vi "test_DL120115FPGA.vi"() -> ()   [LabVIEW 2010, in "FPGAWrapperDL090211Galvo_grabber.lvclass"]
uses:
  FPGAWrapperDL090211Galvo_grabber.lvclass
  common_typedefs/channels_cluster.ctl
  common_typedefs/gate_parameters_cluster.ctl
  common/classes/ErrorController/ErrorController/ErrorController.lvclass
  common/classes/ErrorController/ErrorController/class_data.vi
panel:
  in  "triggered?":bool
  out "samples read":i32
  in  "gate 1 settings":T1
  in  "channel offsets":T2
  out "error controller loaded?":bool=TRUE
  out "pixel dwell time":dbl[unit]
  out "timed out?":bool
  in  "timeout (ms)":i32=500
  out "DAQ loop counter":i32
  out "channel data block":dbl[][](graph)
  in  "number of channels":i32=3
  in  "block size":i32=10000
  out "DL090211FPGAWrapper out":refnum<class "FPGAWrapperDL090211Galvo_grabber.lvclass">
  in  "number of pixels":i64=1000000000
  in  "iterations per pixel":i32=250
  in  "run button":bool
  in  "stop":bool
  in  "create button":bool
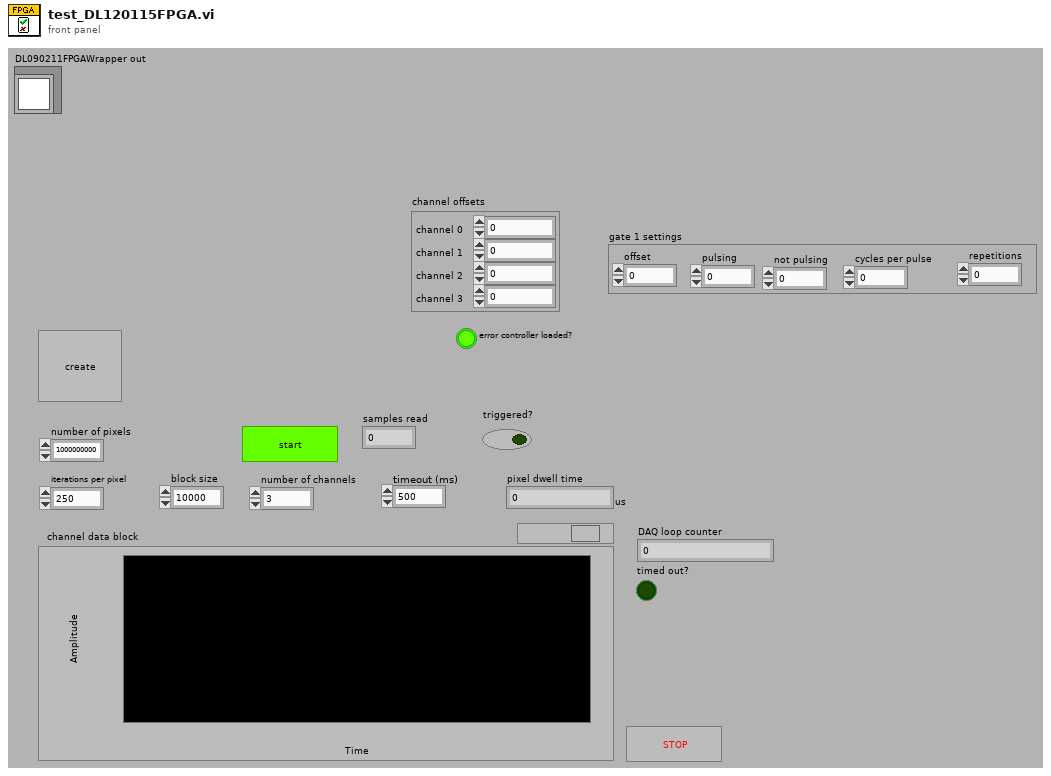
[diagram p1: front panel]
types:
  T1 = typedef "gate_parameters_cluster.ctl" = cluster{"offset":i64, "pulsing":i64, "not pulsing":i64, "cycles per pulse":i64, "repetitions":i64}
  T2 = typedef "channels_cluster.ctl" = cluster{"channel 0":u32, "channel 1":u32, "channel 2":u32, "channel 3":u32}
  T3 = typedef "pixel_raw_data_array.ctl" = dbl[][]
  T4 = typedef "plugin_specification.ctl" = cluster{"class path":string, "configuration":string, "label":string, "settings name":string}
  T5 = typedef "XComponentSpecification.xctl/data.ctl" = cluster{"class path":string, "configuration":string, "label":string, "settings name":string}
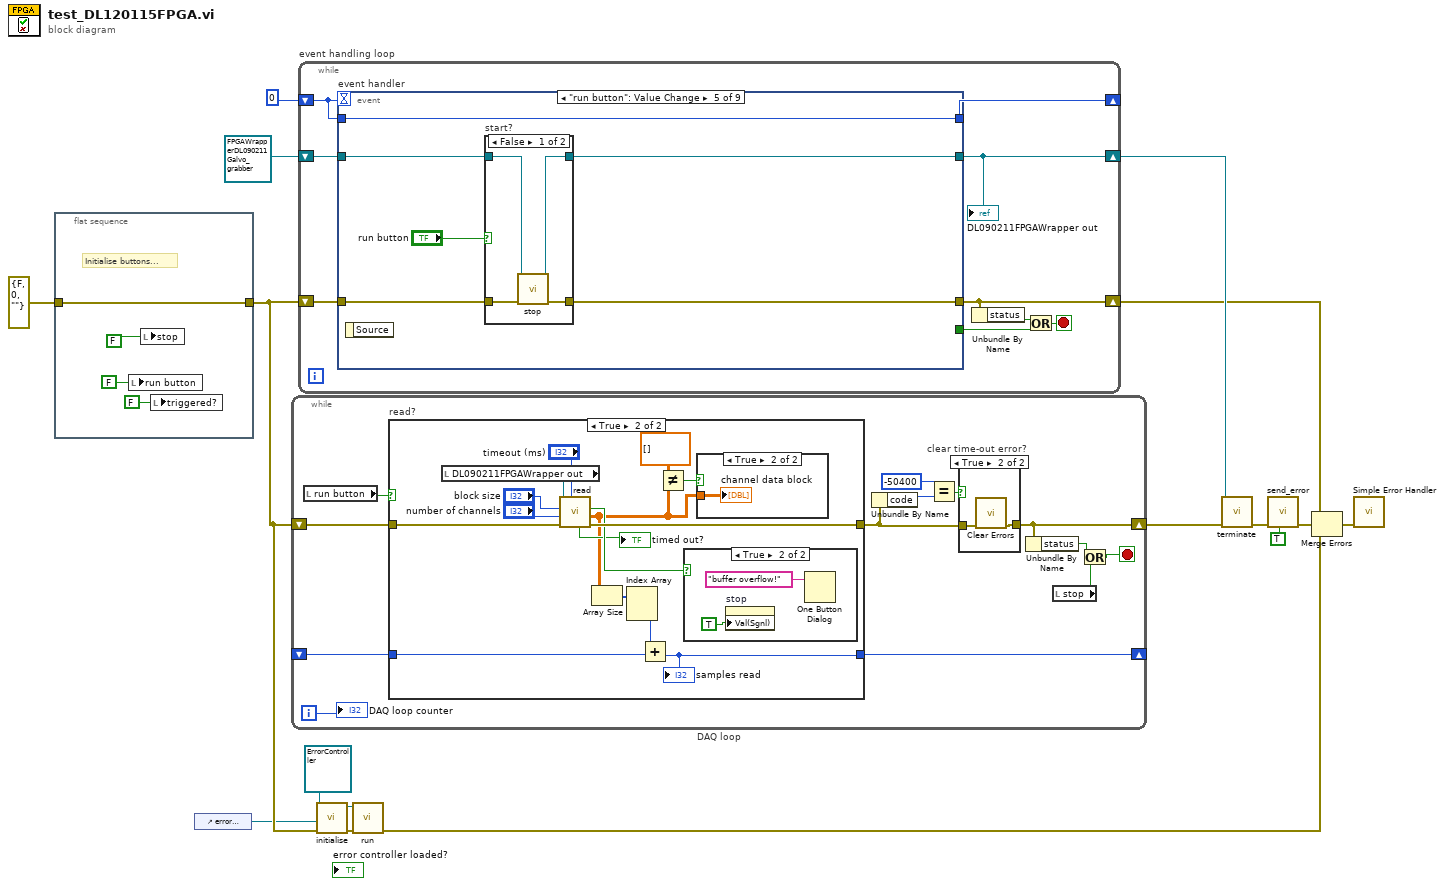
[diagram p0: block diagram]
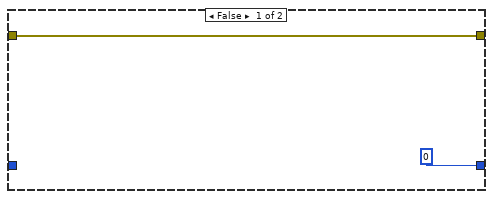
[diagram p3: hidden frame]
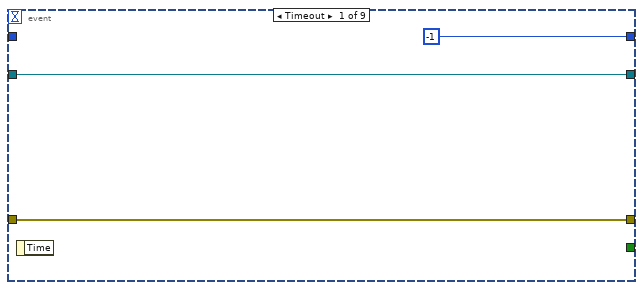
[diagram p6: hidden frame]
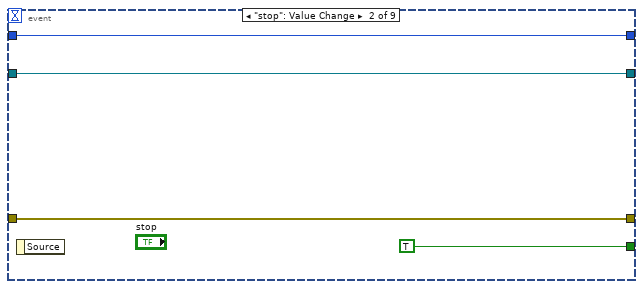
[diagram p7: hidden frame]
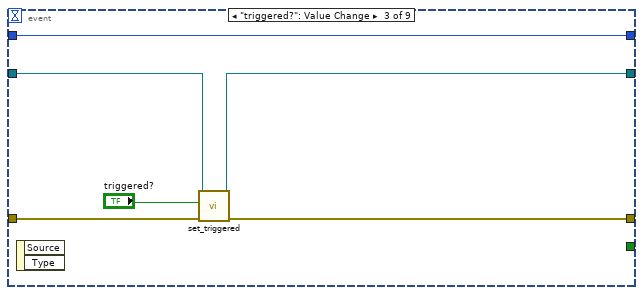
[diagram p8: hidden frame]
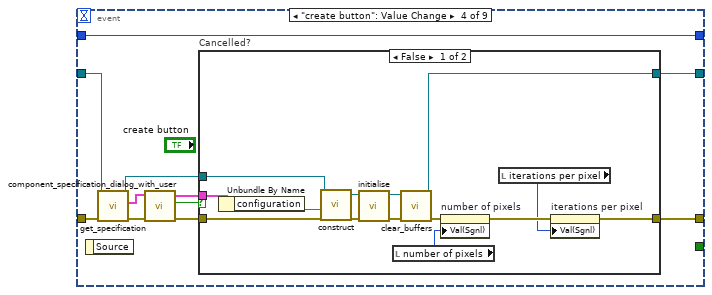
[diagram p9: hidden frame]
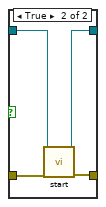
[diagram p11: hidden frame]
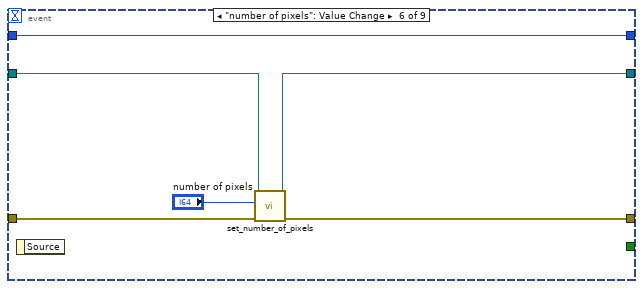
[diagram p12: hidden frame]
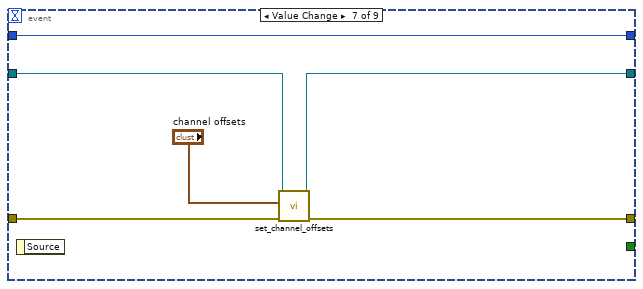
[diagram p13: hidden frame]
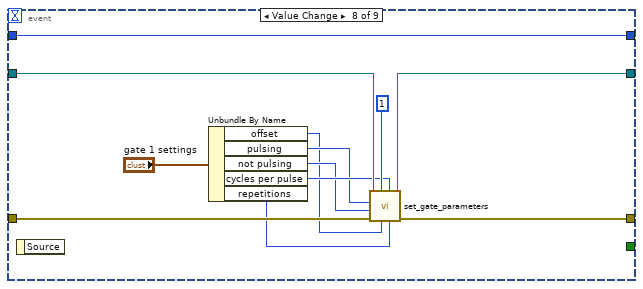
[diagram p14: hidden frame]
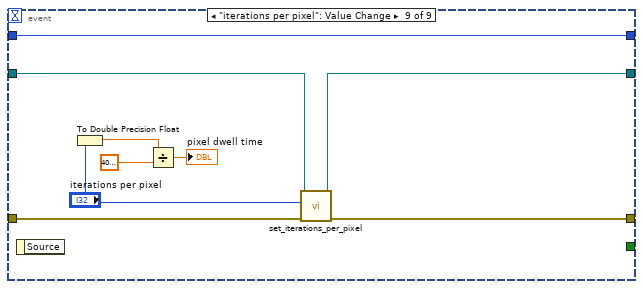
[diagram p15: hidden frame]
diagram:
  n1 = flat-sequence {
    tunnel: errorcluster {"status"=FALSE, "code"=0, "source"=""} ("error in (no error)") -> [w20]
    tunnel: [w20] -> w6
    frame #0 {
      # "Initialise buttons..."
      n2 = local write "run button"(FALSE ("run button")) -> ()
      n3 = local write "stop"(FALSE) -> ()
      n4 = local write "triggered?"(FALSE ("triggered?")) -> ()
    }
  }
  n5 = control-ref of="error controller loaded?"() -> (w1:refnum<vi>)
  n6 = while "DAQ loop" {
    shift-right: [w27] -> w13
    shift-left: w6 -> [w33]
    shift-right: [w21] -> _
    shift-left: _ -> [w22]
    i -> [w23]
    stop <- w24 stop-if-true
    n7 = local read "run button"() -> (w32:bool)
    n8 = case "read?" shown="True" w32 {
      tunnel: w33 -> [w38 w53]
      tunnel: [w38 w52] -> w29
      tunnel: w22 -> [_ w43]
      tunnel: [0 w40] -> w21
      frame False {
      }
      frame True {
        n9 = local read "DL090211FPGAWrapper out"() -> (w51:refnum<class "FPGAWrapperDL090211Galvo_grabber.lvclass">)
        n10 = call-dynamic "read.vi"("timeout (ms)"="timeout (ms)", "error in (no error)"=w53, "number of channels"="number of channels", "block size"="block size", "FPGAWrapperDL090211Galvo in"=w51) -> ("error out"=w52:errorcluster, "channels raw data block"=w42:T3, "FIFO full?"=w46:bool, "timed out?"=→"timed out?":bool)  [unwired: 3 out]
        n11 = Array Size(array=w42) -> (size(s)=w41:i32[])
        n12 = Index Array(array=w41) -> (element #2=w39:i32)  [unwired: 2 in, 1 out]
        n13 = Add(x=w39, y=w43) -> (x+y=w40:i32)
        "samples read" <- w40
        n14 = Not Equal?(x=dbl[][] [], y=w42) -> (x != y?=w48:bool)
        n15 = case shown="True" w46 {
          frame False {
          }
          frame True {
            n16 = property on="stop" class="Bool (strict)"("Val(Sgnl)"=TRUE) -> ()  [unwired: 2 in, 2 out]
            n17 = One Button Dialog(message="buffer overflow!") -> ()  [unwired: 1 in, 1 out]
          }
        }
        n18 = case shown="True" w48 {
          tunnel: w42 -> [_ w56]
          frame False {
          }
          frame True {
            "channel data block" <- w56
          }
        }
      }
    }
    n19 = Unbundle By Name(w29) -> ("code"=w31:i32)
    n20 = Equal?(x=-50400, y=w31) -> (x = y?=w28:bool)
    n21 = case "clear time-out error?" shown="True" w28 {
      tunnel: w29 -> [w34 w36]
      tunnel: [w34 w35] -> w27
      frame False {
      }
      frame True {
        n22 = call <vilib>:"Clear Errors.vi"("error in (no error)"=w36) -> ("error out"=w35:errorcluster)  [unwired: 6 out]
      }
    }
    n23 = Unbundle By Name(w27) -> ("status"=w26:bool)
    n24 = local read "stop"() -> (w25:bool)
    n25 = Or(x=w26, y=w25) -> (x .or. y?=w24:bool)
    "DAQ loop counter" <- w23
  }
  n26 = while "event handling loop" {
    shift-right: [w60] -> w11
    shift-left: w6 -> [w65]
    shift-right: [w63] -> _
    shift-left: 0 -> [w64]
    shift-right: [w61] -> w12
    shift-left: refnum<class "FPGAWrapperDL090211Galvo_grabber.lvclass"> refnum ("DL090211FPGAWrapper.lvclass") -> [w62]
    stop <- w57 stop-if-true
    n27 = event "event handler" shown="[4] \"run button\": Value Change" {
      selector: _ -> [_ _ _ _ _ _ _ _ _]
      dyn-events: _ -> [_ _ _ _ _ _ _ _ _]
      timeout: w64 -> [_ _ _ _ _ _ _ _ _]
      tunnel: [w66 w69 w76 w88 w107 w123 w129 w141 w150] -> w60
      tunnel: w65 -> [w66 w69 w77 w85 w110 w124 w130 w142 w151]
      tunnel: w64 -> [_ w72 w78 w89 w111 w125 w131 w143 w152]
      tunnel: [-1 w72 w78 w89 w111 w125 w131 w143 w152] -> w63
      tunnel: [_ TRUE _ _ _ _ _ _ _] -> w58
      tunnel: [w67 w70 w74 w80 w108 w121 w126 w139 w148] -> w61
      tunnel: w62 -> [w67 w70 w75 w83 w109 w122 w127 w140 w149]
      event Timeout {
        n28 = event-data() -> ()  [unwired: 2 out]
      }
      event "stop": Value Change {
        n29 = event-data() -> ()  [unwired: 2 out]
      }
      event "triggered?": Value Change {
        n30 = event-data() -> ()  [unwired: 3 out]
        n31 = call-dynamic "set_triggered.vi"("error in (no error)"=w77, "triggered?"="triggered?", "FPGAWrapperDL090211Galvo in"=w75) -> ("error out"=w76:errorcluster, "FPGAWrapperDL090211Galvo out"=w74:refnum<class "FPGAWrapperDL090211Galvo_grabber.lvclass">)  [unwired: 7 in]
      }
      event "create button": Value Change {
        n32 = event-data() -> ()  [unwired: 2 out]
        n33 = call-dynamic "get_specification.vi"("error in (no error)"=w85, "GenericPlugin in"=w83) -> ("error out"=w84:errorcluster, "component specification"=w81:T4, "GenericPlugin out"=w82:refnum<class "FPGAWrapperDL090211Galvo_grabber.lvclass">)  [unwired: 6 in, 1 out]
        n34 = call "component_specification_dialog_with_user.vi"("error in (no error)"=w84, "component specification in"=w81) -> ("error out"=w87:errorcluster, "cancelled?"=w79:bool, "component specification out"=w86:T5)  [unwired: 7 in]
        n35 = case "Cancelled?" shown="False" w79 {
          tunnel: [w100 w105] -> w88
          tunnel: w87 -> [w94 w105]
          tunnel: w86 -> [w93 _]
          tunnel: w82 -> [w91 w104]
          tunnel: [w90 w104] -> w80
          frame False {
            n36 = Unbundle By Name(w93) -> ("configuration"=w92:string)
            n37 = call-dynamic "construct.vi"("error in (no error)"=w94, "configuration name"=w92, "GenericPlugin in"=w91) -> ("error out"=w96:errorcluster, "GenericPlugin out"=w95:refnum<class "FPGAWrapperDL090211Galvo_grabber.lvclass">)  [unwired: 7 in]
            n38 = call-dynamic "initialise.vi"("error in (no error)"=w96, "GenericPlugin in"=w95) -> ("error out"=w99:errorcluster, "GenericPlugin out"=w97:refnum<class "FPGAWrapperDL090211Galvo_grabber.lvclass">)  [unwired: 1 in, 7 out]
            n39 = local read "number of pixels"() -> (w101:i64)
            n40 = call-dynamic "clear_buffers.vi"("error in (no error)"=w99, "FPGAWrapperDL090211Galvo in"=w97) -> ("error out"=w98:errorcluster, "FPGAWrapperDL090211Galvo out"=w90:refnum<class "FPGAWrapperDL090211Galvo_grabber.lvclass">)  [unwired: 8 in]
            n41 = property on="number of pixels" class="DigNum (strict)"(error in=w98, "Val(Sgnl)"=w101) -> (error out=w103:errorcluster)  [unwired: 1 in, 1 out]
            n42 = local read "iterations per pixel"() -> (w102:i32)
            n43 = property on="iterations per pixel" class="DigNum (strict)"(error in=w103, "Val(Sgnl)"=w102) -> (error out=w100:errorcluster)  [unwired: 1 in, 1 out]
          }
          frame True {
          }
        }
      }
      event "run button": Value Change {
        n44 = event-data() -> ()  [unwired: 2 out]
        n45 = case "start?" shown="False" "run button" {
          tunnel: w110 -> [w115 w119]
          tunnel: w109 -> [w113 w118]
          tunnel: [w112 w117] -> w108
          tunnel: [w114 w116] -> w107
          frame False {
            n46 = call-dynamic "stop.vi"("error in (no error)"=w115, "FPGAWrapperDL090211Galvo in"=w113) -> ("error out"=w114:errorcluster, "FPGAWrapperDL090211Galvo out"=w112:refnum<class "FPGAWrapperDL090211Galvo_grabber.lvclass">)  [unwired: 8 out]
          }
          frame True {
            n47 = call-dynamic "start.vi"("error in (no error)"=w119, "FPGAWrapperDL090211Galvo in"=w118) -> ("error out"=w116:errorcluster, "FPGAWrapperDL090211Galvo out"=w117:refnum<class "FPGAWrapperDL090211Galvo_grabber.lvclass">)  [unwired: 8 out]
          }
        }
      }
      event "number of pixels": Value Change {
        n48 = event-data() -> ()  [unwired: 2 out]
        n49 = call-dynamic "set_number_of_pixels.vi"("error in (no error)"=w124, "number of pixels"="number of pixels", "FPGAWrapperDL090211Galvo in"=w122) -> ("error out"=w123:errorcluster, "FPGAWrapperDL090211Galvo out"=w121:refnum<class "FPGAWrapperDL090211Galvo_grabber.lvclass">)  [unwired: 7 out]
      }
      event Value Change {
        n50 = event-data() -> ()  [unwired: 2 out]
        n51 = call-dynamic "set_channel_offsets.vi"("error in (no error)"=w130, "pixel values cluster"="channel offsets", "FPGAWrapperDL090211Galvo in"=w127) -> ("error out"=w129:errorcluster, "FPGAWrapperDL090211Galvo out"=w126:refnum<class "FPGAWrapperDL090211Galvo_grabber.lvclass">)  [unwired: 7 in]
      }
      event Value Change {
        n52 = event-data() -> ()  [unwired: 2 out]
        n53 = Unbundle By Name("gate 1 settings") -> ("offset"=w133:i64, "pulsing"=w135:i64, "not pulsing"=w134:i64, "cycles per pulse"=w136:i64, "repetitions"=w132:i64)
        n54 = call-dynamic "set_gate_parameters.vi"("repetitions"=w132, "pulse duration (iterations)"=w136, "offset duration (iterations)"=w133, "clock index"=1, "error in (no error)"=w142, "low phase duration (iterations)"=w134, "high phase duration (iterations)"=w135, "FPGAWrapperDL090211Galvo in"=w140) -> ("error out"=w141:errorcluster, "FPGAWrapperDL090211Galvo out"=w139:refnum<class "FPGAWrapperDL090211Galvo_grabber.lvclass">)  [unwired: 2 in]
      }
      event "iterations per pixel": Value Change {
        n55 = event-data() -> ()  [unwired: 2 out]
        n56 = To Double Precision Float(number="iterations per pixel") -> (double precision float=w146:dbl)
        n57 = Divide(x=w146, y=dbl[unit] 40000000.0) -> (x/y=→"pixel dwell time":dbl[unit])
        n58 = call-dynamic "set_iterations_per_pixel.vi"("error in (no error)"=w151, "iterations per pixel"="iterations per pixel", "FPGAWrapperDL090211Galvo in"=w149) -> ("error out"=w150:errorcluster, "FPGAWrapperDL090211Galvo out"=w148:refnum<class "FPGAWrapperDL090211Galvo_grabber.lvclass">)  [unwired: 7 out]
      }
    }
    "DL090211FPGAWrapper out" <- w61
    n59 = Unbundle By Name(w60) -> ("status"=w59:bool)
    n60 = Or(x=w59, y=w58) -> (x .or. y?=w57:bool)
  }
  n61 = call-dynamic "initialise.vi"("error in (no error)"=w6, "error boolean"=w1, "ErrorController in"=refnum<class "ErrorController.lvclass"> refnum) -> ("error out"=w9:errorcluster, "ErrorController out"=w8:refnum<class "ErrorController.lvclass">)  [unwired: 7 in]
  n62 = call "run.vi"("error in (no error)"=w9, "ErrorController in"=w8) -> ("error out"=w2:errorcluster)  [unwired: 8 in, 1 out]
  n63 = call-dynamic "terminate.vi"("error in (no error)"=w13, "GenericPlugin in"=w12) -> ("error out"=w5:errorcluster)  [unwired: 9 out]
  n64 = call "send_error.vi"("last error? (F)"=TRUE, "error in (no error)"=w5) -> ("error out"=w4:errorcluster)  [unwired: 9 in]
  n65 = Merge Errors(w11, w4, w2) -> (w10:errorcluster)
  n66 = call <vilib>:"Simple Error Handler.vi"("error in (no error)"=w10) -> ()  [unwired: 1 in, 8 out]
